vi "test collection.vi"() -> ()   [LabVIEW 2013, in "tag bus tests.lvlib"]
uses:
  tag bus tests.lvlib
  tag/tag descriptor.lvclass/tag descriptor.ctl
  tag collection/tag collection.lvclass
  tag/tag descriptor.lvclass
panel:
  out "found all 2":bool
  out "found all":bool
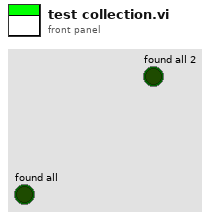
[diagram p1: front panel]
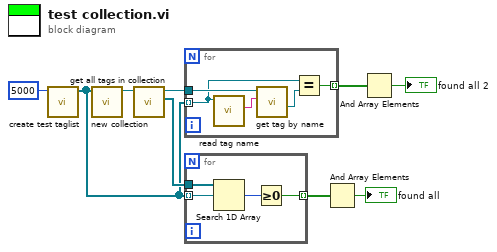
[diagram p0: block diagram]
diagram:
  n1 = call "create test taglist.vi"("count"=5000) -> ("tags"=w4:refnum<class "tag descriptor.lvclass">[])  [unwired: 7 in, 3 out]
  n2 = call "new collection.vi"("tags"=w4) -> ("tag collection out"=w9:refnum<class "tag collection.lvclass">)  [unwired: 9 in, 1 out]
  n3 = call "get all tags in collection.vi"("tag collection in"=w9) -> ("tags"=w8:refnum<class "tag descriptor.lvclass">[], "tag collection out"=w5:refnum<class "tag collection.lvclass">)  [unwired: 8 in, 1 out]
  n4 = for {
    tunnel: w5 -> [w14]
    tunnel: w4 -> [w11] mode=indexing
    tunnel: [w10] -> w2 mode=indexing
    n5 = call "read tag name.vi"("system tag in"=w11) -> ("name"=w13:string)  [unwired: 8 in, 2 out]
    n6 = call "get tag by name.vi"("tag"=w13, "tag collection in"=w14) -> ("located tag"=w12:refnum<class "tag descriptor.lvclass">)  [unwired: 7 in, 2 out]
    n7 = Equal?(x=w11, y=w12) -> (x = y?=w10:bool)
  }
  n8 = for {
    tunnel: w8 -> [w18]
    tunnel: w4 -> [w17] mode=indexing
    tunnel: [w15] -> w7 mode=indexing
    n9 = Search 1D Array(1D array=w18, element=w17) -> (index of element=w16:i32)  [unwired: 1 in]
    n10 = Greater Or Equal To 0?(x=w16) -> (x >= 0?=w15:bool)
  }
  n11 = And Array Elements(Boolean array=w7) -> (logical AND=→"found all":bool)
  n12 = And Array Elements(Boolean array=w2) -> (logical AND=→"found all 2":bool)
